vi "user process.vi"(8 "error in":errorcluster, 11 "Parameters to process":T2) -> (0 "error out":errorcluster, 3 "Results from processing":T1)   [LabVIEW 2013, in "Temperature Controller Logic runtime.lvclass"]
doc: "This functionality implements PID control for the lamp, and converts the Fan Boolean into a 0-100 duty cycle."
uses:
  Temperature Controller Logic runtime.lvclass
  parameter user data.ctl
  result user data.ctl
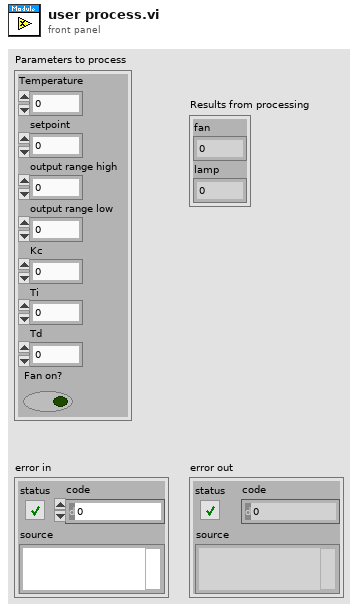
[diagram p1: front panel]
types:
  T1 = typedef "Temperature Controller Logic runtime.lvclass/result user data.ctl" = cluster{"fan":dbl, "lamp":dbl}
  T2 = typedef "Temperature Controller Logic runtime.lvclass/parameter user data.ctl" = cluster{"Temperature":dbl, "setpoint":dbl, "output range high":dbl, "output range low":dbl, "Kc":dbl, "Ti":dbl, "Td":dbl, "Fan on?":bool}
  T3 = cluster{"proportional gain (Kc)":dbl, "integral time (Ti, min)":dbl, "derivative time (Td, min)":dbl}
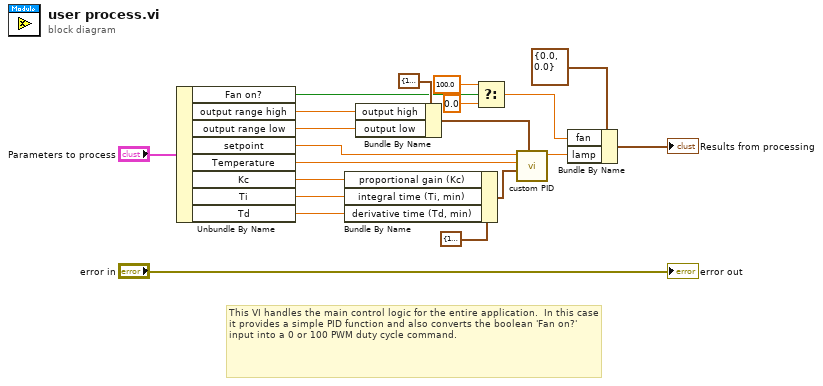
[diagram p0: block diagram]
diagram:
  # "This VI handles the main control logic for the entire application.  In this case it provides a simple PID function and also converts the boolean 'Fan on?' input into a 0 or 100 PWM duty cycle command."
  n1 = Unbundle By Name("Parameters to process") -> ("Fan on?"=w9:bool, "output range high"=w14:dbl, "output range low"=w16:dbl, "setpoint"=w4:dbl, "Temperature"=w3:dbl, "Kc"=w12:dbl, "Ti"=w11:dbl, "Td"=w10:dbl)
  n2 = Bundle By Name(cluster=T3 {"proportional gain (Kc)"=1.0, "integral time (Ti, min)"=0.01, "derivative time (Td, min)"=0.0} ("PID gains"), "proportional gain (Kc)"=w12, "integral time (Ti, min)"=w11, "derivative time (Td, min)"=w10) -> (w2:T3)
  n3 = Bundle By Name(cluster=cluster{"output high":dbl, "output low":dbl} {"output high"=100.0, "output low"=0.0} ("output range"), "output high"=w14, "output low"=w16) -> (w5:cluster{"output high":dbl, "output low":dbl})
  n4 = Select(t=100.0, s=w9, f=0.0) -> (s? t:f=w6:dbl)
  n5 = call "custom PID.vi"("output range"=w5, "PID gains"=w2, "process variable"=w3, "setpoint"=w4) -> ("output"=w1:dbl)  [unwired: 6 in, 1 out]
  n6 = Bundle By Name(cluster=T1 {"fan"=0.0, "lamp"=0.0} ("Results from processing"), "fan"=w6, "lamp"=w1) -> (→"Results from processing":T1)
  "error out" <- "error in"
